vi "Load DevInfo From File.vi"(8 "error in (no error)":errorcluster, 11 "Controller in":refnum<class "Controller.lvclass">) -> (0 "error out":errorcluster, 3 "Controller out":refnum<class "Controller.lvclass">)   [LabVIEW 2016]
uses:
  <userlib>/Common Components/Controller/Controller.lvclass
  <userlib>/Common Components/Controller UI/Update DT event data.ctl
  <userlib>/Common Components/Controller UI/Update DT Cmd.ctl
  <userlib>/Common Components/Controller UI Messages/Update DT Event Msg/Update DT Event Msg.lvclass/Update DT Event Msg.ctl
  <vilib>/ActorFramework/Message Enqueuer/Message Enqueuer.lvclass/Message Enqueuer.ctl
  <vilib>/ActorFramework/Message Enqueuer/Enqueue.vi
  <userlib>/Common Components/Controller UI Messages/Update DT Event Msg/Update DT Event Msg.lvclass
  C:/Program Files (x86)/National Instruments/LabVIEW 2016/vi.lib/ActorFramework/Message/Message.lvclass
  <vilib>/ActorFramework/Message Priority Queue/Priority Enqueue.vi
  <userlib>/Common Components/Controller UI/Controller UI.lvclass
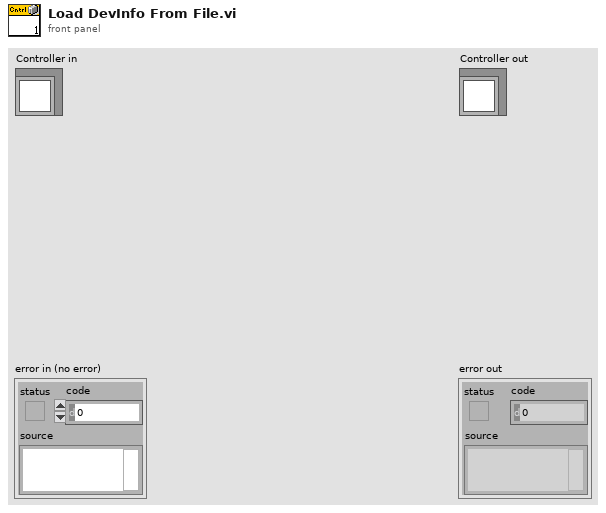
[diagram p1: front panel]
types:
  T1 = typedef "Controller UI.lvlib/Controller UI.lvclass/Update DT event data.ctl" = cluster{"Cmd":T2, "Data Array":variant[]}
  T2 = typedef "Controller UI.lvlib/Controller UI.lvclass/Update DT Cmd.ctl" = enum16{"Update HWtype\\HWplugin array", "Update Checked-out", "Update COMM Status", "Load DevInfo from File", "Save DevInfo to File"}
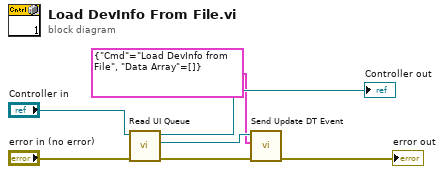
[diagram p0: block diagram]
diagram:
  n1 = call <userlib>:"Read UI Queue.vi"("error in (no error)"="error in (no error)", "UI Controller in"="Controller in") -> ("error out"=w6:errorcluster, "UI Queue"=w2:refnum<class "Message Enqueuer.lvclass">, "UI Controller out"=→"Controller out":refnum<class "Controller.lvclass">)  [unwired: 7 in]
  n2 = call <userlib>:"Send Update DT Event.vi"("error in (no error)"=w6, "event data"=T1 {"Cmd"=enum."Load DevInfo from File", "Data Array"=[]}, "Message Enqueuer"=w2) -> ("error out"=→"error out":errorcluster)  [unwired: 7 in, 1 out]
